vi "queryConfig.vi"(0 "连接ID":refnum<k5>, 1 "item":string(combo)="config") -> (2 "连接ID输出":refnum<k5>, 3 "x":dbl, 4 "y":dbl, 5 "z":dbl)   [LabVIEW 2017]
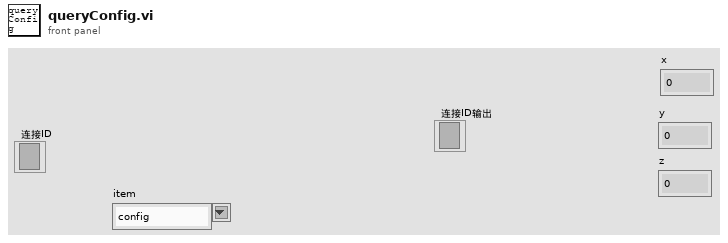
[diagram p1: front panel]
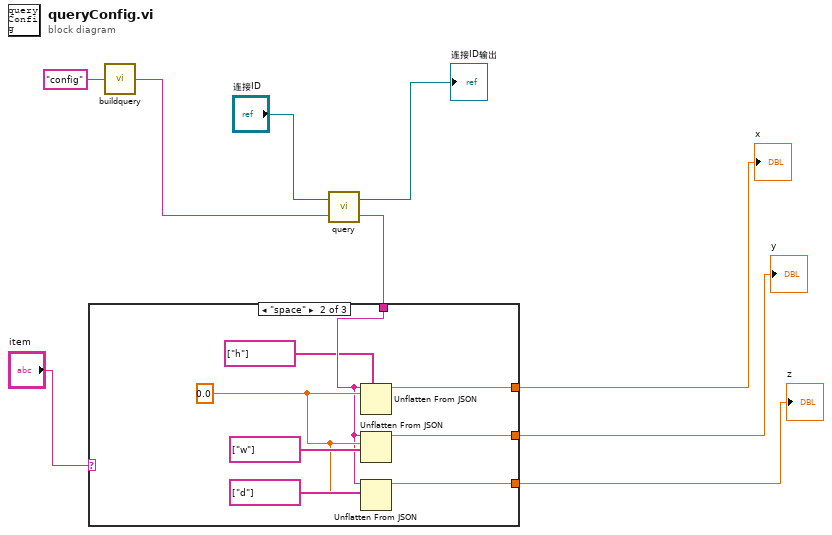
[diagram p0: block diagram]
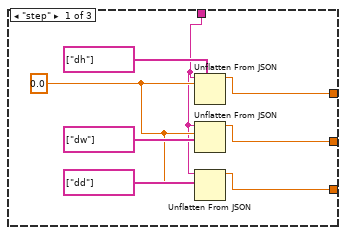
[diagram p2: hidden frame]
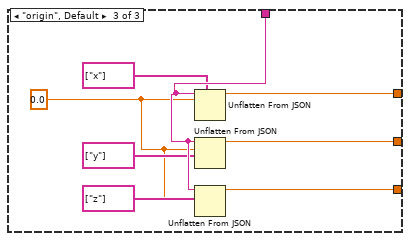
[diagram p3: hidden frame]
diagram:
  n1 = call "buildquery.vi"("String"="config") -> ("JSON字符串"=w5:string)
  n2 = call "query.vi"("数据输入"=w5, "连接ID"="连接ID") -> ("数据输出"=w4:string, "连接ID输出"=→"连接ID输出":refnum<k5>)
  n3 = case shown="\"space\"" "item" {
    tunnel: w4 -> [w12 w22 w33]
    tunnel: [w13 w20 w28] -> w3
    tunnel: [w11 w19 w27] -> w2
    tunnel: [w10 w18 w26] -> w1
    frame "step" {
      w14 = 0.0 ("z 2")
      n4 = Unflatten From JSON(path=string[] ["dh"] ("路径"), JSON string=w12, type and defaults=w14) -> (value=w13:dbl)  [unwired: 4 in, 1 out]
      n5 = Unflatten From JSON(path=string[] ["dw"] ("路径"), JSON string=w12, type and defaults=w14) -> (value=w11:dbl)  [unwired: 4 in, 1 out]
      n6 = Unflatten From JSON(path=string[] ["dd"] ("路径"), JSON string=w12, type and defaults=w14) -> (value=w10:dbl)  [unwired: 4 in, 1 out]
    }
    frame "space" {
      w23 = 0.0 ("z 2")
      n7 = Unflatten From JSON(path=string[] ["h"] ("路径"), JSON string=w22, type and defaults=w23) -> (value=w20:dbl)  [unwired: 4 in, 1 out]
      n8 = Unflatten From JSON(path=string[] ["w"] ("路径"), JSON string=w22, type and defaults=w23) -> (value=w19:dbl)  [unwired: 4 in, 1 out]
      n9 = Unflatten From JSON(path=string[] ["d"] ("路径"), JSON string=w22, type and defaults=w23) -> (value=w18:dbl)  [unwired: 4 in, 1 out]
    }
    frame "origin", Default {
      w29 = 0.0 ("z 2")
      n10 = Unflatten From JSON(path=string[] ["x"] ("路径"), JSON string=w33, type and defaults=w29) -> (value=w28:dbl)  [unwired: 4 in, 1 out]
      n11 = Unflatten From JSON(path=string[] ["y"] ("路径"), JSON string=w33, type and defaults=w29) -> (value=w27:dbl)  [unwired: 4 in, 1 out]
      n12 = Unflatten From JSON(path=string[] ["z"] ("路径"), JSON string=w33, type and defaults=w29) -> (value=w26:dbl)  [unwired: 4 in, 1 out]
    }
  }
  "x" <- w3
  "y" <- w2
  "z" <- w1
